vi "Monitor Report Value.vi"(8 "error in":errorcluster, 11 "DataIn":T1={"State"=enum."APU Select", "2D User Info"=[], "APU Setup File"={"Sensor Info"=[], "Variables"=[], "CMM Table 106"=[], "CMM Table 106B "=[], "Accel Config"=[], "Report Sheet 1"=[], "Report Sheet 2"=[], "Report Sheet 3"=[]}, "Test Information"={"APU Part Number:"="", "Model:"="", "Serial Number:"="", "Customer:"="", "Work Order:"="", "Pre or Post SB"="", "Run Count"=0, "APU Selected"="<Select>"}, "ChannelTags"=[], "Live_Min_Max_Dev"=[], "CalChannels"=[], "Slopes"=[], "Offsets"=[], "Calculated Values"={"C.00"=0.0, "C.01"=0.0, "C.02"=0.0, "C.03"=0.0, "C.04"=0.0, "C.05"=0.0, "C.06"=0.0, "C.07"=0.0, "C.08"=0.0, "C.09"=0.0, "C.10"=0.0, "C.11"=0.0, "C.12"=0.0, "C.13"=0.0, "C.14"=0.0, "C.15"=0.0, "C.16"=0.0, "C.17"=0.0, "C.18"=0.0, "C.19"=0.0, "C.20"=0.0, "C.21"=0.0, "C.22"=0.0, "C.23"=0.0, "C.24"=0.0, "C.25"=0.0, "C.26"=0.0, "C.27"=0.0, "C.28"=0.0, "C.29"=0.0, "C.30"=0.0, "C.31"=0.0, "C.32"=0.0, "C.33"=0.0, "C.34"=0.0, "C.35"=0.0, "C.36"=0.0, "C.37"=0.0, "C.38"=0.0, "C.39"=0.0, "C.40"=0.0, "C.41"=0.0, "C.42"=0.0, "C.43"=0.0, "C.44"=0.0, "C.45"=0.0, "C.46"=0.0, "C.47"=0.0, "C.48"=0.0, "C.49"=0.0, "C.50"=0.0, "C.51"=0.0, "C.52"=0.0, "C.53"=0.0, "C.54"=0.0, "C.55"=0.0, "C.56"=0.0, "C.57"=0.0, "C.58"=0.0, "C.59"=0.0, "C.60"=0.0, "C.61"=0.0, "C.62"=0.0}, "ThresholdChannels"=[], "ThresholdRPM"=[], "ThresholdMin"=[], "ThresholdValue"=[], "HeavyCCM"=[], "LightCCM"=[], "FuelFarm"=FALSE} {"Test Information"."Run Count" min=0 step=1}) -> (0 "error out":errorcluster, 3 "DataOut":T1={"State"=enum."APU Select", "2D User Info"=[], "APU Setup File"={"Sensor Info"=[], "Variables"=[], "CMM Table 106"=[], "CMM Table 106B "=[], "Accel Config"=[], "Report Sheet 1"=[], "Report Sheet 2"=[], "Report Sheet 3"=[]}, "Test Information"={"APU Part Number:"="", "Model:"="", "Serial Number:"="", "Customer:"="", "Work Order:"="", "Pre or Post SB"="", "Run Count"=0, "APU Selected"="<Select>"}, "ChannelTags"=[], "Live_Min_Max_Dev"=[], "CalChannels"=[], "Slopes"=[], "Offsets"=[], "Calculated Values"={"C.00"=0.0, "C.01"=0.0, "C.02"=0.0, "C.03"=0.0, "C.04"=0.0, "C.05"=0.0, "C.06"=0.0, "C.07"=0.0, "C.08"=0.0, "C.09"=0.0, "C.10"=0.0, "C.11"=0.0, "C.12"=0.0, "C.13"=0.0, "C.14"=0.0, "C.15"=0.0, "C.16"=0.0, "C.17"=0.0, "C.18"=0.0, "C.19"=0.0, "C.20"=0.0, "C.21"=0.0, "C.22"=0.0, "C.23"=0.0, "C.24"=0.0, "C.25"=0.0, "C.26"=0.0, "C.27"=0.0, "C.28"=0.0, "C.29"=0.0, "C.30"=0.0, "C.31"=0.0, "C.32"=0.0, "C.33"=0.0, "C.34"=0.0, "C.35"=0.0, "C.36"=0.0, "C.37"=0.0, "C.38"=0.0, "C.39"=0.0, "C.40"=0.0, "C.41"=0.0, "C.42"=0.0, "C.43"=0.0, "C.44"=0.0, "C.45"=0.0, "C.46"=0.0, "C.47"=0.0, "C.48"=0.0, "C.49"=0.0, "C.50"=0.0, "C.51"=0.0, "C.52"=0.0, "C.53"=0.0, "C.54"=0.0, "C.55"=0.0, "C.56"=0.0, "C.57"=0.0, "C.58"=0.0, "C.59"=0.0, "C.60"=0.0, "C.61"=0.0, "C.62"=0.0}, "ThresholdChannels"=[], "ThresholdRPM"=[], "ThresholdMin"=[], "ThresholdValue"=[], "HeavyCCM"=[], "LightCCM"=[], "FuelFarm"=FALSE} {"Test Information"."Run Count" min=0 step=1})   [LabVIEW 2018, in "Controller (Host).lvlib"]
uses:
  Controller (Host).lvlib
  Private Controls/Controller (Host) Data.ctl
  Private Controls/State.ctl
  Top Level/Shared Controls/APU Setup File.ctl
  Public Controls/Test Information.ctl
  Public VIs/PreorPostSB.ctl
  Public Controls/APU Select.ctl
  Top Level/Shared Controls/Calculated Data.ctl
  Testing UI 1/Testing UI 1.lvlib
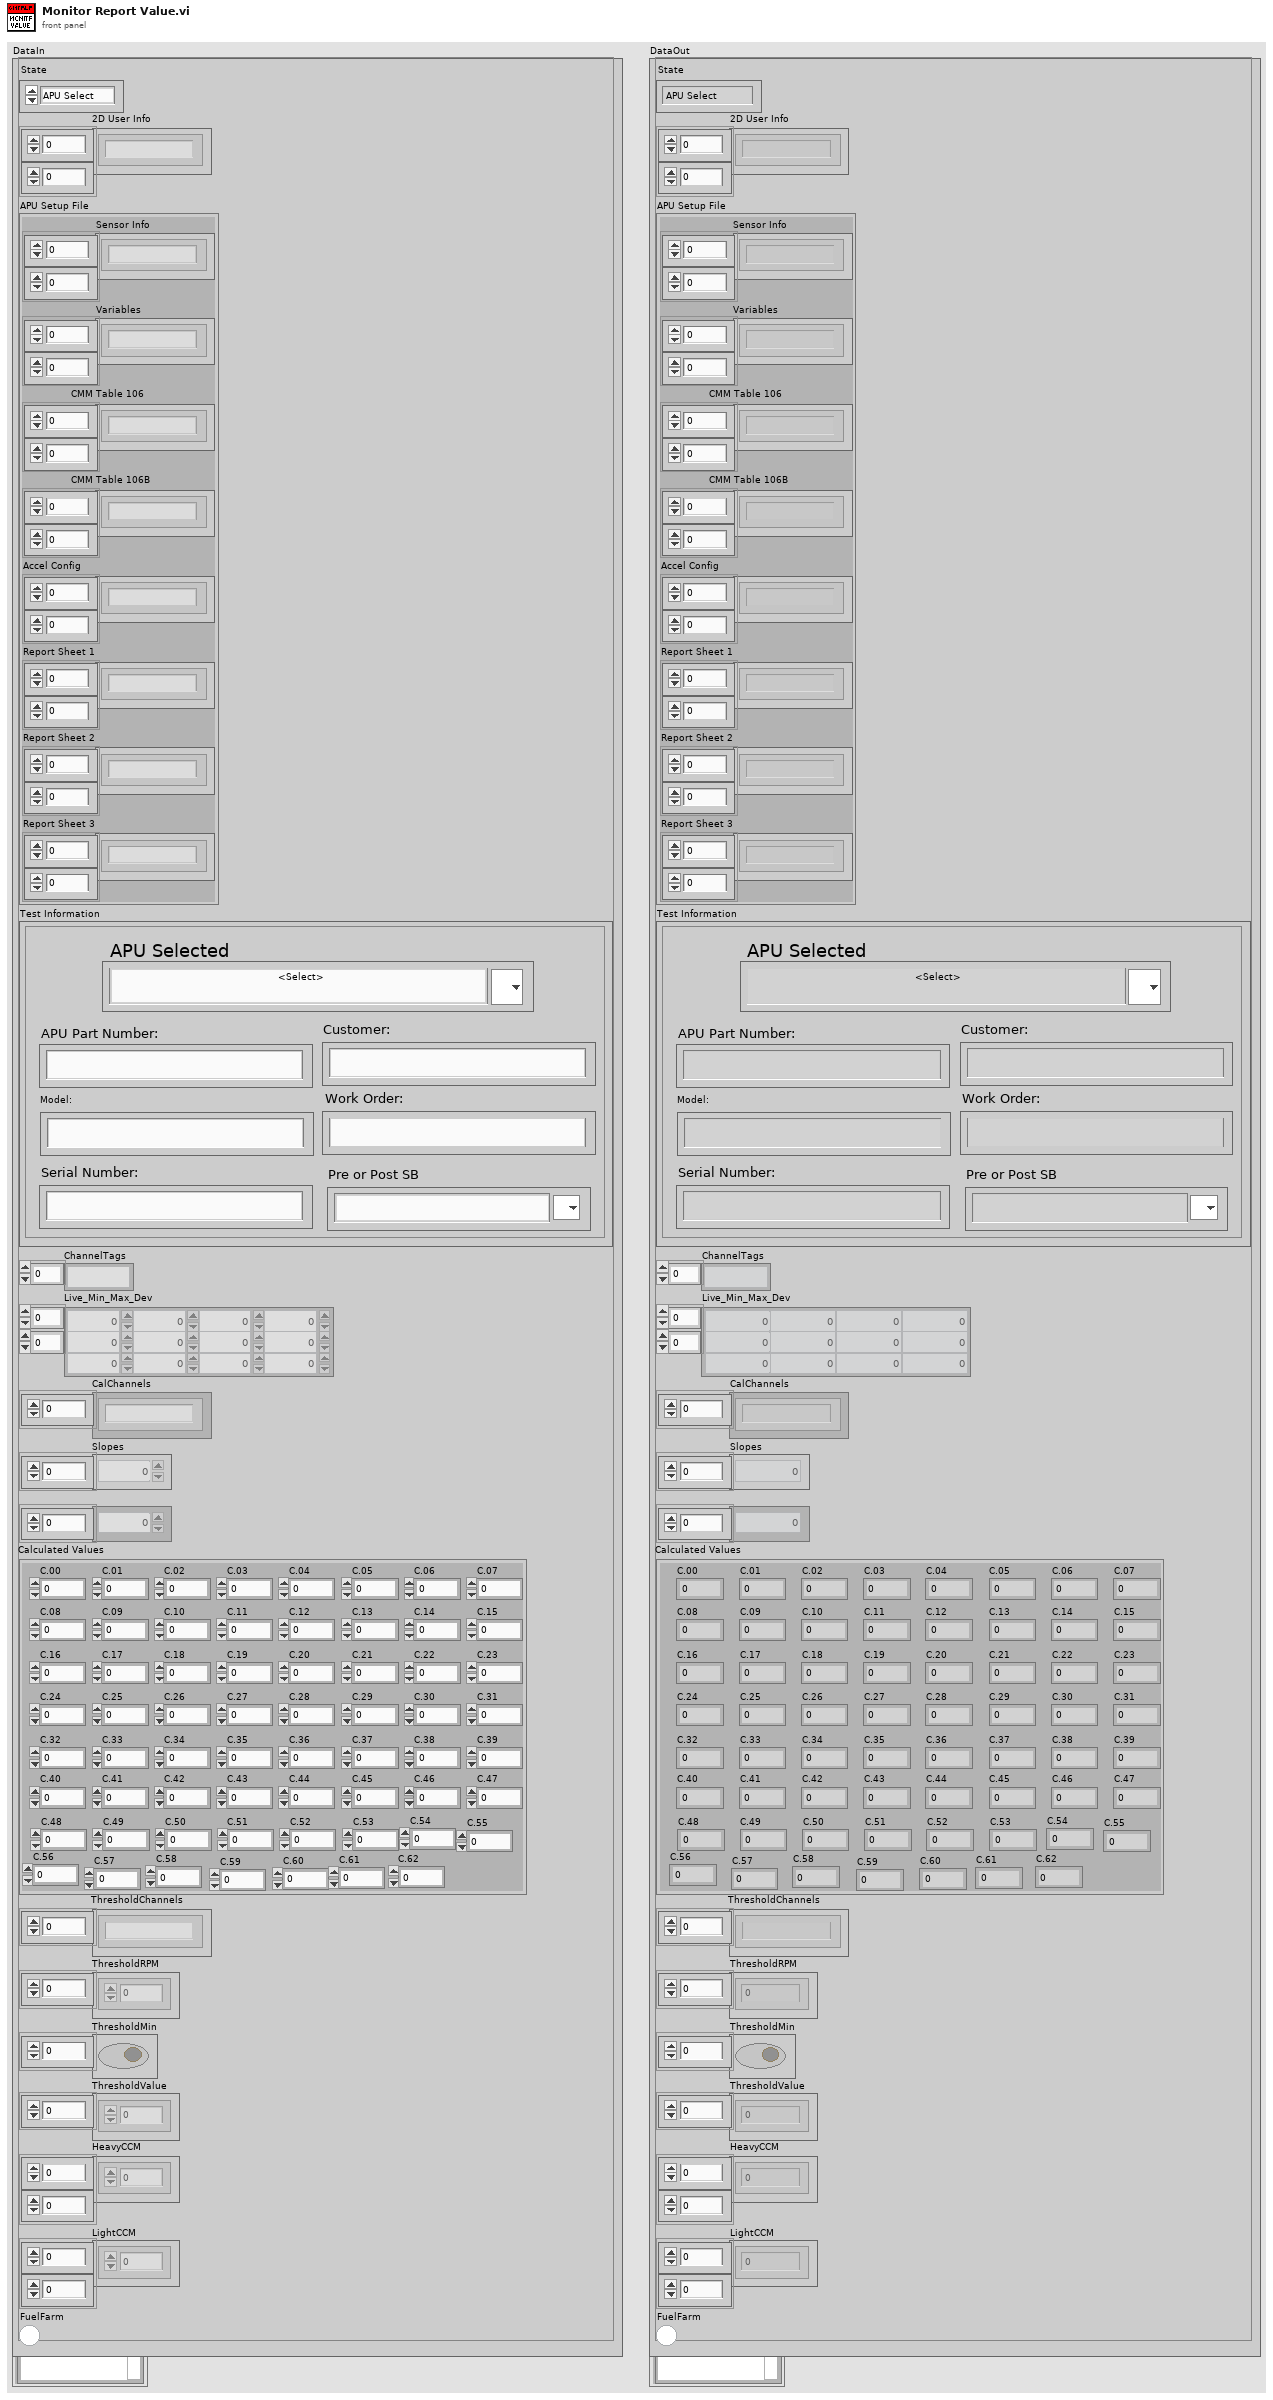
[diagram p1: front panel]
types:
  T1 = typedef "Controller (Host).lvlib/Controller (Host) Data.ctl" = cluster{"State":T2, "2D User Info":string[][], "APU Setup File":T3, "Test Information":T4, "ChannelTags":string[], "Live_Min_Max_Dev":dbl[][], "CalChannels":string[], "Slopes":dbl[], "Offsets":dbl[], "Calculated Values":T7, "ThresholdChannels":string[], "ThresholdRPM":dbl[], "ThresholdMin":bool[], "ThresholdValue":dbl[], "HeavyCCM":dbl[][], "LightCCM":dbl[][], "FuelFarm":bool}
  T2 = typedef "Controller (Host).lvlib/State.ctl" = enum16{"APU Select", "Operation Select", "SubTests Select", "Calibration", "Testing", "Exit"}
  T3 = typedef "APU Setup File.ctl" = cluster{"Sensor Info":string[][], "Variables":string[][], "CMM Table 106":string[][], "CMM Table 106B ":string[][], "Accel Config":string[][], "Report Sheet 1":string[][], "Report Sheet 2":string[][], "Report Sheet 3":string[][]}
  T4 = typedef "Controller (Host).lvlib/Test Information.ctl" = cluster{"APU Part Number:":string, "Model:":string, "Serial Number:":string, "Customer:":string, "Work Order:":string, "Pre or Post SB":T5, "Run Count":i32, "APU Selected":T6}
  T5 = typedef "Controller (Host).lvlib/PreorPostSB.ctl" = string
  T6 = typedef "Controller (Host).lvlib/APU Select.ctl" = string
  T7 = typedef "Calculated Data.ctl" = cluster{"C.00":dbl, "C.01":dbl, "C.02":dbl, "C.03":dbl, "C.04":dbl, "C.05":dbl, "C.06":dbl, "C.07":dbl, "C.08":dbl, "C.09":dbl, "C.10":dbl, "C.11":dbl, "C.12":dbl, "C.13":dbl, "C.14":dbl, "C.15":dbl, "C.16":dbl, "C.17":dbl, "C.18":dbl, "C.19":dbl, "C.20":dbl, "C.21":dbl, "C.22":dbl, "C.23":dbl, "C.24":dbl, "C.25":dbl, "C.26":dbl, "C.27":dbl, "C.28":dbl, "C.29":dbl, "C.30":dbl, "C.31":dbl, "C.32":dbl, "C.33":dbl, "C.34":dbl, "C.35":dbl, "C.36":dbl, "C.37":dbl, "C.38":dbl, "C.39":dbl, "C.40":dbl, "C.41":dbl, "C.42":dbl, "C.43":dbl, "C.44":dbl, "C.45":dbl, "C.46":dbl, "C.47":dbl, "C.48":dbl, "C.49":dbl, "C.50":dbl, "C.51":dbl, "C.52":dbl, "C.53":dbl, "C.54":dbl, "C.55":dbl, "C.56":dbl, "C.57":dbl, "C.58":dbl, "C.59":dbl, "C.60":dbl, "C.61":dbl, "C.62":dbl}
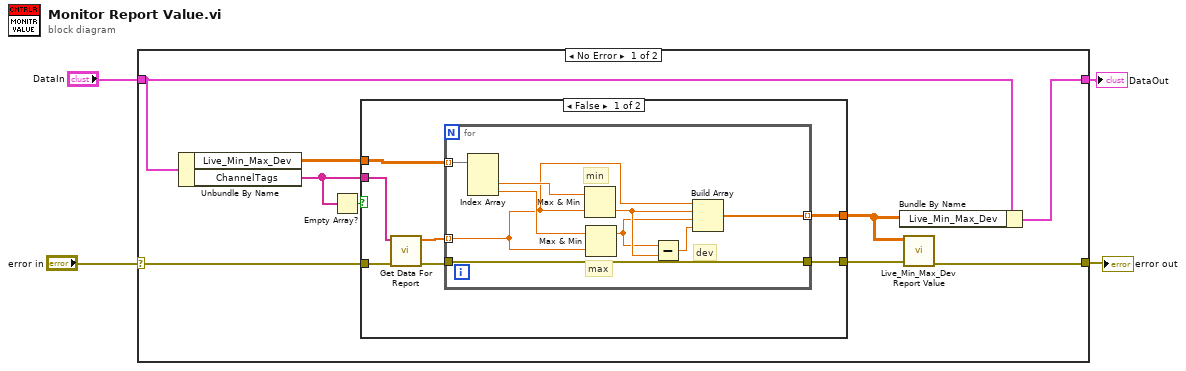
[diagram p0: block diagram]
diagram:
  n1 = case shown="No Error" "error in" {
    selector: "error in" -> [w12 w33]
    tunnel: "DataIn" -> [w11 w32]
    tunnel: [w10 w32] -> w2
    tunnel: [w8 w33] -> w4
    frame No Error {
      n2 = Unbundle By Name(w11) -> ("Live_Min_Max_Dev"=w13:dbl[][], "ChannelTags"=w6:string[])
      n3 = Empty Array?(array=w6) -> (empty?=w5:bool)
      n4 = case shown="False" w5 {
        tunnel: w13 -> [w20 w30]
        tunnel: w12 -> [w17 w31]
        tunnel: [w19 w31] -> w9
        tunnel: [w18 w30] -> w7
        tunnel: w6 -> [w15 _]
        frame False {
          n5 = call "Get Data For Report.vi"("error constant"=w17, "Channel Tags"=w15) -> ("error out"=w16:errorcluster, "Value"=w14:dbl[])  [unwired: 8 in]
          n6 = for {
            tunnel: w20 -> [w29] mode=indexing
            tunnel: [w28] -> w18 mode=indexing
            tunnel: w16 -> [w27]
            tunnel: [w27] -> w19
            tunnel: w14 -> [w21] mode=indexing
            # "dev"
            # "max"
            # "min"
            n7 = Index Array(array=w29) -> (element #2=w26:dbl, element #3=w25:dbl)  [unwired: 3 in, 1 out]
            n8 = Max & Min(x=w26, y=w21) -> (min(x,y)=w24:dbl)  [unwired: 1 out]
            n9 = Max & Min(x=w25, y=w21) -> (max(x,y)=w23:dbl)  [unwired: 1 out]
            n10 = Subtract(x=w23, y=w24) -> (x-y=w22:dbl)
            n11 = Build Array(w21, w24, w23, w22) -> (w28:dbl[])
          }
        }
        frame True {
        }
      }
      n12 = Bundle By Name(cluster=w11, "Live_Min_Max_Dev"=w7) -> (w10:T1)
      n13 = call "Live_Min_Max_Dev Report Value.vi"("error in (no error)"=w9, "Live, Min, Max, Dev"=w7) -> ("error out"=w8:errorcluster)  [unwired: 9 in]
    }
    frame Error {
    }
  }
  "error out" <- w4
  "DataOut" <- w2
